vi "private_iterator.vi"() -> (3 "iterator":u32)   [LabVIEW 2013, in "Caraya.lvlib"]
uses:
  Caraya.lvlib
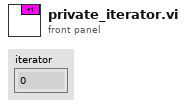
[diagram p1: front panel]
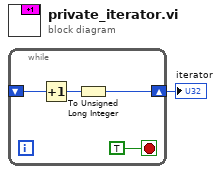
[diagram p0: block diagram]
diagram:
  n1 = while {
    shift-right: [w3] -> w1
    shift-left: _ -> [w5]
    stop <- TRUE stop-if-true
    n2 = Increment(x=w5) -> (x+1=w4:u32)
    n3 = To Unsigned Long Integer(number=w4) -> (unsigned 32bit integer=w3:u32)
  }
  "iterator" <- w1
